vi "ForceSettings3D.vi"(9 "Function":i32) -> (1 "k":dbl format="%#_13g", 2 "Setpoint":dbl format="%#_13g")   [LabVIEW 2023]
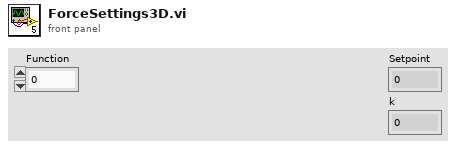
[diagram p1: front panel]
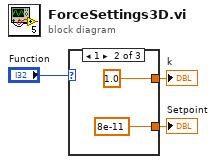
[diagram p0: block diagram]
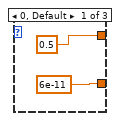
[diagram p2: hidden frame]
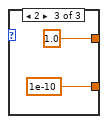
[diagram p3: hidden frame]
diagram:
  n1 = case shown="1" "Function" {
    tunnel: [0.5 1.0 1.0] -> w2
    tunnel: [6e-11 8e-11 1e-10] -> w1
    frame 0, Default {
    }
    frame 1 {
    }
    frame 2 {
    }
  }
  "Setpoint" <- w1
  "k" <- w2
